vi "SbigOpenSynchronization.vi"(2 "Sbig List":string[](array[string]), 9 "error in (no error)":errorcluster) -> (0 "Command Queue out":T2, 6 "error out":errorcluster, 7 "Notifiers out":T1[](array[typedef]))   [LabVIEW 2009]
uses:
  Controls/SbigCommandQueue.ctl
  Controls/SbigCommand.ctl
  Controls/SbigStatusNotifier.ctl
  Controls/SbigStatus.ctl
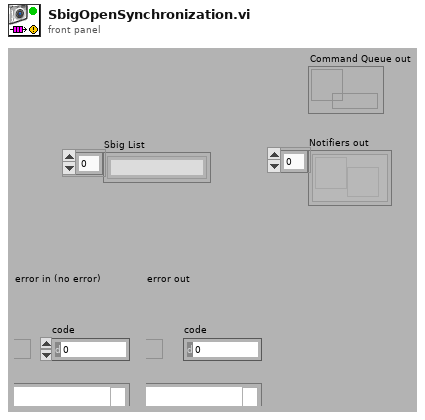
[diagram p1: front panel]
types:
  T1 = typedef "SbigStatusNotifier.ctl" = refnum<notifier>
  T2 = typedef "SbigCommandQueue.ctl" = refnum<queue>
  T3 = typedef "SbigCommand.ctl" = cluster{"Sbig":string, "Command":enum16{"EXPOSE", "SET TEMP", "SET MISC", "QUIT"}, "Time":u32, "Window":cluster{"X0":u16, "Y0":u16, "DX":u16, "DY":u16, "on/off":bool}, "Temp":cluster{"Regulation":u16, "Auto Freeze":u16, "CCD Set Point":dbl}, "Misc":cluster{"Fan":u16, "Shutter":u16, "Led":u16}}
  T4 = typedef "SbigStatus.ctl" = cluster{"Managed ?":bool, "State":enum16{"IDLE", "EXPOSING", "READING"}, "Image":i32[][], "Temperature Info":cluster{"Temperature Regulation":bool, "T Setpoint":dbl, "T CCD":dbl, "T Ambient":dbl, "Cooling %":dbl}}
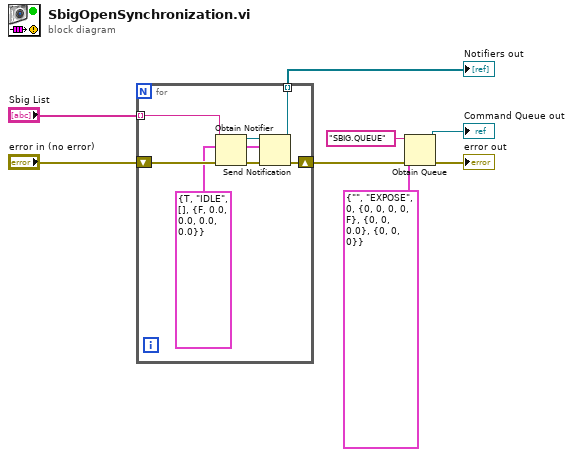
[diagram p0: block diagram]
diagram:
  n1 = for {
    shift-right: [w12] -> w4
    shift-left: "error in (no error)" -> [w15]
    tunnel: [w13] -> w1 mode=indexing
    tunnel: "Sbig List" -> [w10] mode=indexing
    w9 = T4 {"Managed ?"=TRUE, "State"=enum."IDLE", "Image"=[], "Temperature Info"={"Temperature Regulation"=FALSE, "T Setpoint"=0.0, "T CCD"=0.0, "T Ambient"=0.0, "Cooling %"=0.0}} ("Axis Status")
    n2 = Obtain Notifier(name (unnamed)=w10, notification data type=w9, error in (no error)=w15) -> (notifier out=w11:refnum<notifier>, error out=w14:errorcluster)  [unwired: 1 in, 1 out]
    n3 = Send Notification(notification=w9, notifier=w11, error in (no error)=w14) -> (notifier out=w13:refnum<notifier>, error out=w12:errorcluster)
  }
  "Notifiers out" <- w1
  n4 = Obtain Queue(name (unnamed)="SBIG.QUEUE" ("nom (aucun)"), element data type=T3 {"Sbig"="", "Command"=enum."EXPOSE", "Time"=0, "Window"={"X0"=0, "Y0"=0, "DX"=0, "DY"=0, "on/off"=FALSE}, "Temp"={"Regulation"=0, "Auto Freeze"=0, "CCD Set Point"=0.0}, "Misc"={"Fan"=0, "Shutter"=0, "Led"=0}} ("SbigCommand"), error in (no error)=w4) -> (queue out=→"Command Queue out":refnum<queue>, error out=→"error out":errorcluster)  [unwired: 2 in, 1 out]
